vi "Get or Add Cell.vi"(8 "error in":errorcluster, 10 "Cell Address":string, 11 "Worksheetpart in":refnum<k24>) -> (0 "error out":errorcluster, 2 "Cell":refnum<k24>, 3 "WorksheetPart out":refnum<k24>)   [LabVIEW 2021, in "Open Xml.lvlib"]
uses:
  Open Xml.lvlib
  D:/git/Open-Xml-LabVIEW/dll/DocumentFormat.OpenXml.dll
  dll/DocumentFormat.OpenXml.dll
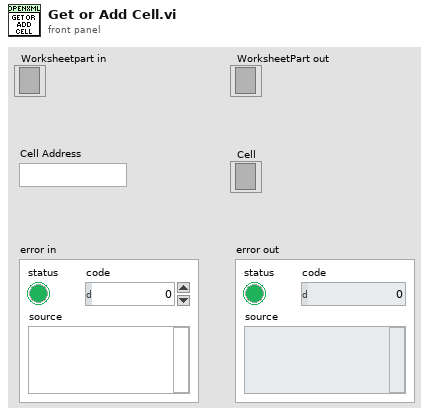
[diagram p1: front panel]
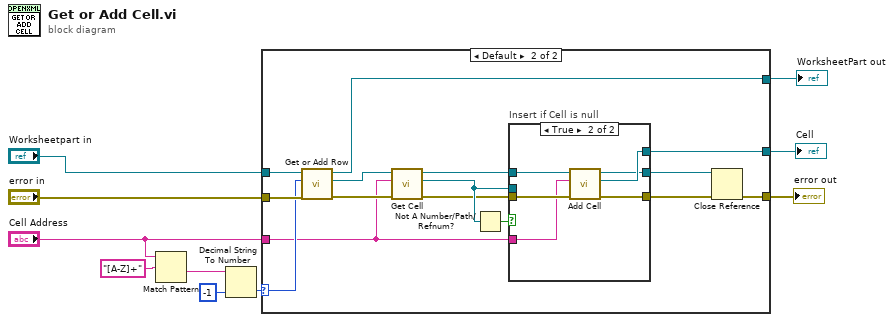
[diagram p0: block diagram]
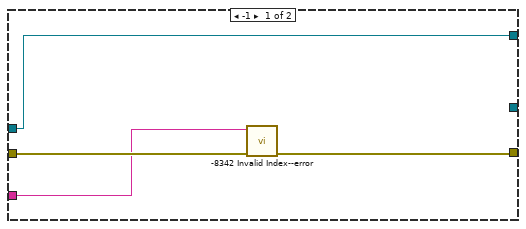
[diagram p2: hidden frame]
diagram:
  n1 = Match Pattern(string="Cell Address", regular expression="[A-Z]+") -> (after substring=w6:string)  [unwired: 1 in, 3 out]
  n2 = Decimal String To Number(string=w6, default (0L)=i64 -1 ("default (0 I32)")) -> (number=w4:i64)  [unwired: 1 in, 1 out]
  n3 = case shown="Default" w4 {
    selector: w4 -> [_ w25]
    tunnel: [_ w28] -> w10
    tunnel: "error in" -> [w14 w27]
    tunnel: "Worksheetpart in" -> [w11 w26]
    tunnel: [w11 w21] -> w3
    tunnel: "Cell Address" -> [w12 w18]
    tunnel: [w13 w16] -> w1
    frame -1 {
      n4 = call "-8342 Invalid Index--error.vi"("error in"=w14, "Index"=w12) -> ("error out"=w13:errorcluster)  [unwired: 9 in]
    }
    frame Default {
      n5 = call "Get or Add Row.vi"("error in"=w27, "Row Index"=w25, "Worksheetpart in"=w26) -> ("error out"=w23:errorcluster, "Row"=w24:refnum<k24>, "WorksheetPart out"=w21:refnum<k24>)  [unwired: 6 in]
      n6 = call "Get Cell.vi"("error in"=w23, "Cell Address"=w18, "Row in"=w24) -> ("error out"=w20:errorcluster, "Cell"=w22:refnum<k24>, "Row out"=w19:refnum<k24>)  [unwired: 6 in]
      n7 = Not A Number/Path/Refnum?(number/path/refnum=w22) -> (NaN/Path/Refnum?=w29:bool)
      n8 = case "Insert if Cell is null" shown="True" w29 {
        tunnel: w20 -> [w32 w38]
        tunnel: [w32 w37] -> w17
        tunnel: [w31 w34] -> w28
        tunnel: w22 -> [w31 _]
        tunnel: w19 -> [w30 w36]
        tunnel: w18 -> [_ w35]
        tunnel: [w30 w33] -> w15
        frame False {
        }
        frame True {
          n9 = call "Add Cell.vi"("error in"=w38, "Cell Address"=w35, "Row in"=w36) -> ("error out"=w37:errorcluster, "Cell"=w34:refnum<k24>, "Row out"=w33:refnum<k24>)  [unwired: 6 in]
        }
      }
      n10 = Close Reference(reference=w15, error in (no error)=w17) -> (error out=w16:errorcluster)
    }
  }
  "error out" <- w1
  "Cell" <- w10
  "WorksheetPart out" <- w3
